vi "SeCrTs-RT_Sequence_Main.vi"(8 "error in":errorcluster) -> (0 "error out":errorcluster)   [LabVIEW 2022 SP3]
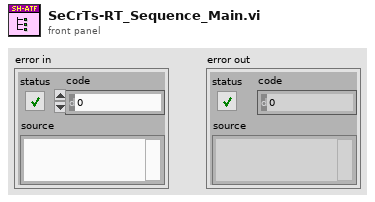
[diagram p1: front panel]
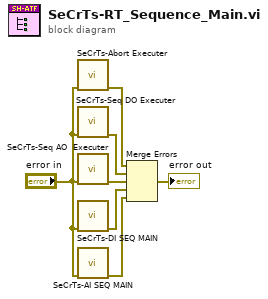
[diagram p0: block diagram]
diagram:
  n1 = call "SeCrTs-Abort Executer.vi"("error in"="error in") -> ("error IO"=w1:errorcluster)  [unwired: 10 in]
  n2 = call "SeCrTs-Seq DO Executer .vi"("error in"="error in") -> ("error IO"=w7:errorcluster)  [unwired: 10 in]
  n3 = call "SeCrTs-Seq AO  Executer.vi"("error in"="error in") -> ("error IO"=w6:errorcluster)  [unwired: 10 in]
  n4 = call "SeCrTs-DI SEQ MAIN.vi"("error in"="error in") -> ("error Out"=w5:errorcluster)  [unwired: 10 in]
  n5 = call "SeCrTs-AI SEQ MAIN.vi"("error IO"="error in") -> ("error Out"=w4:errorcluster)  [unwired: 10 in]
  n6 = Merge Errors(w1, w7, w6, w5, w4) -> (→"error out":errorcluster)
